vi "PH_Beamline.i attribute.vi"(0 "VI Refnum":refnum<vi>, 2 "CLASS.i attribute":T1={"GUI Refs"={"PA ok"=refnum, "MA ok"=refnum, "fs FE ok"=refnum, "ns FE ok"=refnum, "PA ED ok"=refnum, "MAS ok"=refnum, "Booster ok"=refnum, "Mirrortower ok"=refnum, "In.-Box ok"=refnum, "Compressor ok"=refnum, "Experiment LB ok"=refnum, "Experiment LL ok"=refnum, "PHELIX_Beckhoff_Watchdog"=refnum, "Shutters closed"=refnum, "uOPA ok"=refnum, "Vacuum no shotcond Comp LB"=refnum}, "Refs BL MA"=[], "Refs BL MA-IB"=[], "Refs BL fs"=[], "Refs BL PA ED"=[], "Refs BL MAS"=[], "Refs BL Boo"=[], "Refs BL ns"=[], "Refs BL Mirrortower"=[], "Refs BL Compressor"=[], "Refs BL Exp LB"=[], "Radiation Safety"={"Exp Laserbay"={"Ref Op Mode"=refnum, "Ref Laserbay evacuated"=refnum, "Tagname LB evacuated"="N/A", "Shot Mode"=0, "Laserbay evacuated?"=0, "Tagname HV room locked"="N/A", "HV room locked?"=0, "Ref HV room locked"=refnum, "Tagname bridged?"="N/A", "Ref Bridge"=refnum, "I<1E18W/cm²"=FALSE}, "Exp Laserlab"={"Ref Op Mode"=refnum, "Ref Laserlab evacuated"=refnum, "Tagname LL evacuated"="N/A", "Shot Mode"=0, "Laserlab evacuated?"=0, "Tagname bridged?"="N/A", "Ref Bridge"=refnum, "I<1E18W/cm²"=FALSE}}, "Refs BL LL"=[], "PP Igni Heating GUI Refs"=[], "PP Igni Heating Tagnames "=[], "Refs BL PA"={"undelayed Line before Shutter"=[], "undelayed Line after Shutter"=[], "before Bypass"=[], "delayed Line before Shutter"=[], "delayed Line after Shutter"=[], "before Shutter Input"=[], "after Shutter Input"=[], "Bypass"=[], "before Shutter Exit"=[], "after Shutter Exit"=[], "to MA"=[], "to Lab"=[]}, "BL"={"YLF_BL_Status"=-1, "fs_BL_Status"=-1, "fs_YLF_BL_Status"=-1, "ns_BL_Status"=-1, "PA_Input_BL_Status"=-1, "PA_UnDelay_BL_Status"=-1, "PA_Delay_BL_Status"=-1, "PA_BL_Status"=-1, "PA_Bypass_BL_Status"=-1, "PA_Exit_BL_Status"=-1, "PA_LL_BL_Status"=-1, "LL_BL_Status"=-1, "PA_MA_BL_Status"=-1, "MA_Exit_BL_Status"=-1, "MA_Z6_BL_Status"=-1, "Z6_BL_Status"=-1, "MA_LB_BL_Status"=-1, "LB_TB2_BL_Status"=-1, "PA_before_Bypass_BL_Status"=-1, "LB_TB3_BL_Status"=-1}, "State Subsystems"={"PA"=FALSE, "MA"=FALSE, "ns FE"=FALSE, "fs FE"=FALSE, "PA ED"=FALSE, "In.-Box"=FALSE, "MAS"=FALSE, "Booster"=FALSE, "Mirrortower"=FALSE, "Compressor"=FALSE, "Experiment LB"=FALSE, "Experiment LL"=FALSE, "uOPA"=FALSE}, "Status Subscriber Information"={"fs Swich YLF"={"Index of element"=-1, "Attributeset"=enum."Boolean Status Service Subscriber"}, "fs Exit Shutter"={"Index of element"=-1, "Attributeset"=enum."Boolean Status Service Subscriber"}, "ns Exit Shutter"={"Index of element"=-1, "Attributeset"=enum."Boolean Status Service Subscriber"}, "PA Input Shutter"={"Index of element"=-1, "Attributeset"=enum."Boolean Status Service Subscriber"}, "PA PC WP"={"Index of element"=-1, "Attributeset"=enum."Boolean Status Service Subscriber"}, "PA PC WP 2"={"Index of element"=-1, "Attributeset"=enum."Boolean Status Service Subscriber"}, "PA Bypass In"={"Index of element"=-1, "Attributeset"=enum."Boolean Status Service Subscriber"}, "PA Bypass Out"={"Index of element"=-1, "Attributeset"=enum."Boolean Status Service Subscriber"}, "PA CH 1"={"Index of element"=-1, "Attributeset"=enum."Boolean Status Service Subscriber"}, "PA delayed"={"Index of element"=-1, "Attributeset"=enum."Boolean Status Service Subscriber"}, "PA non delayed"={"Index of element"=-1, "Attributeset"=enum."Boolean Status Service Subscriber"}, "PA Exit Shutter"={"Index of element"=-1, "Attributeset"=enum."Boolean Status Service Subscriber"}, "PA Switch Lab"={"Index of element"=-1, "Attributeset"=enum."Boolean Status Service Subscriber"}, "PA Bridge CH Input MA"={"Index of element"=-1, "Attributeset"=enum."Boolean Status Service Subscriber"}, "MA Diffusor IB"={"Index of element"=-1, "Attributeset"=enum."Boolean Status Service Subscriber"}, "MA IB Ready"={"Index of element"=-1, "Attributeset"=enum."Boolean Status Service Subscriber"}, "MA CH 1"={"Index of element"=-1, "Attributeset"=enum."Boolean Status Service Subscriber"}, "MA CH 2"={"Index of element"=-1, "Attributeset"=enum."Boolean Status Service Subscriber"}, "MA CH 3"={"Index of element"=-1, "Attributeset"=enum."Boolean Status Service Subscriber"}, "MA CH 4"={"Index of element"=-1, "Attributeset"=enum."Boolean Status Service Subscriber"}, "MA Shutter Align Cam"={"Index of element"=-1, "Attributeset"=enum."Boolean Status Service Subscriber"}, "MA Position MM5"={"Index of element"=-1, "Attributeset"=enum."Boolean Status Service Subscriber"}, "Calorimeter Switch"={"Index of element"=-1, "Attributeset"=enum."Boolean Status Service Subscriber"}, "BL Z6 CH 9"={"Index of element"=-1, "Attributeset"=enum."Boolean Status Service Subscriber"}, "BL Z6 Beamdump"={"Index of element"=-1, "Attributeset"=enum."Boolean Status Service Subscriber"}, "BL Z6 Shutter"={"Index of element"=-1, "Attributeset"=enum."Boolean Status Service Subscriber"}, "COS Sensitivity Switch"={"Index of element"=-1, "Attributeset"=enum."Boolean Status Service Subscriber"}, "Exp LB Shutter"={"Index of element"=-1, "Attributeset"=enum."Boolean Status Service Subscriber"}, "Exp LB TB 2"={"Index of element"=-1, "Attributeset"=enum."Boolean Status Service Subscriber"}, "Exp LB TB 3"={"Index of element"=-1, "Attributeset"=enum."Boolean Status Service Subscriber"}, "PA LL Input CH"={"Index of element"=-1, "Attributeset"=enum."Boolean Status Service Subscriber"}, "PA LL Output CH"={"Index of element"=-1, "Attributeset"=enum."Boolean Status Service Subscriber"}, "LL Comp Input Shutter"={"Index of element"=-1, "Attributeset"=enum."Boolean Status Service Subscriber"}, "LL Comp Output Shutter"={"Index of element"=-1, "Attributeset"=enum."Boolean Status Service Subscriber"}, "LL Comp FF Shutter"={"Index of element"=-1, "Attributeset"=enum."Boolean Status Service Subscriber"}, "Exp LL Shutter"={"Index of element"=0, "Attributeset"=enum."Boolean Status Service Subscriber"}, "MA IM In IB"={"Index of element"=0, "Attributeset"=enum."Boolean Status Service Subscriber"}, "MA IM Out IB"={"Index of element"=0, "Attributeset"=enum."Boolean Status Service Subscriber"}, "MA DB In IB"={"Index of element"=0, "Attributeset"=enum."Boolean Status Service Subscriber"}, "MA DB Out IB"={"Index of element"=0, "Attributeset"=enum."Boolean Status Service Subscriber"}, "Exp LB Shutter Interlock"={"Index of element"=0, "Attributeset"=enum."Boolean Status Service Subscriber"}, "Exp LL Shutter Interlock"={"Index of element"=0, "Attributeset"=enum."Boolean Status Service Subscriber"}, "MM1 Force Sensor"={"Index of element"=0, "Attributeset"=enum."Boolean Status Service Subscriber"}}, "Refs BL uOPA"=[], "PA_Input_2_Beam_6PWpGUI not linked?"=FALSE, "PA_Input_Delay_6PGUI not linked?"=FALSE, "Settings"={"PA Doublepass Mode"=FALSE, "Compressor Vaccuum LB not relevant"=FALSE, "Windowshutter TB2 not relevant"=FALSE, "Windowshutter TB3 not relevant"=FALSE}} {"Radiation Safety"."Exp Laserlab"."Laserlab evacuated?" items=["no info", "LL not evacuated", "LL evacuated"]; "Radiation Safety"."Exp Laserlab"."Shot Mode" items=["no info", "no Shotmode", "Shotmode"]; "Radiation Safety"."Exp Laserbay"."HV room locked?" items=["no info", "HV room open", "HV room locked"]; "Radiation Safety"."Exp Laserbay"."Laserbay evacuated?" items=["no info", "LB not evacuated", "LB evacuated"]; "Radiation Safety"."Exp Laserbay"."Shot Mode" items=["no info", "no Shotmode", "Shotmode"]}, 3 "Action":T7(ring), 5 "error in (no error)":errorcluster) -> (14 "VI Refnum out":refnum<vi>, 16 "CLASS.i attribute out":T1={"GUI Refs"={"PA ok"=refnum, "MA ok"=refnum, "fs FE ok"=refnum, "ns FE ok"=refnum, "PA ED ok"=refnum, "MAS ok"=refnum, "Booster ok"=refnum, "Mirrortower ok"=refnum, "In.-Box ok"=refnum, "Compressor ok"=refnum, "Experiment LB ok"=refnum, "Experiment LL ok"=refnum, "PHELIX_Beckhoff_Watchdog"=refnum, "Shutters closed"=refnum, "uOPA ok"=refnum, "Vacuum no shotcond Comp LB"=refnum}, "Refs BL MA"=[], "Refs BL MA-IB"=[], "Refs BL fs"=[], "Refs BL PA ED"=[], "Refs BL MAS"=[], "Refs BL Boo"=[], "Refs BL ns"=[], "Refs BL Mirrortower"=[], "Refs BL Compressor"=[], "Refs BL Exp LB"=[], "Radiation Safety"={"Exp Laserbay"={"Ref Op Mode"=refnum, "Ref Laserbay evacuated"=refnum, "Tagname LB evacuated"="N/A", "Shot Mode"=0, "Laserbay evacuated?"=0, "Tagname HV room locked"="N/A", "HV room locked?"=0, "Ref HV room locked"=refnum, "Tagname bridged?"="N/A", "Ref Bridge"=refnum, "I<1E18W/cm²"=FALSE}, "Exp Laserlab"={"Ref Op Mode"=refnum, "Ref Laserlab evacuated"=refnum, "Tagname LL evacuated"="N/A", "Shot Mode"=0, "Laserlab evacuated?"=0, "Tagname bridged?"="N/A", "Ref Bridge"=refnum, "I<1E18W/cm²"=FALSE}}, "Refs BL LL"=[], "PP Igni Heating GUI Refs"=[], "PP Igni Heating Tagnames "=[], "Refs BL PA"={"undelayed Line before Shutter"=[], "undelayed Line after Shutter"=[], "before Bypass"=[], "delayed Line before Shutter"=[], "delayed Line after Shutter"=[], "before Shutter Input"=[], "after Shutter Input"=[], "Bypass"=[], "before Shutter Exit"=[], "after Shutter Exit"=[], "to MA"=[], "to Lab"=[]}, "BL"={"YLF_BL_Status"=-1, "fs_BL_Status"=-1, "fs_YLF_BL_Status"=-1, "ns_BL_Status"=-1, "PA_Input_BL_Status"=-1, "PA_UnDelay_BL_Status"=-1, "PA_Delay_BL_Status"=-1, "PA_BL_Status"=-1, "PA_Bypass_BL_Status"=-1, "PA_Exit_BL_Status"=-1, "PA_LL_BL_Status"=-1, "LL_BL_Status"=-1, "PA_MA_BL_Status"=-1, "MA_Exit_BL_Status"=-1, "MA_Z6_BL_Status"=-1, "Z6_BL_Status"=-1, "MA_LB_BL_Status"=-1, "LB_TB2_BL_Status"=-1, "PA_before_Bypass_BL_Status"=-1, "LB_TB3_BL_Status"=-1}, "State Subsystems"={"PA"=FALSE, "MA"=FALSE, "ns FE"=FALSE, "fs FE"=FALSE, "PA ED"=FALSE, "In.-Box"=FALSE, "MAS"=FALSE, "Booster"=FALSE, "Mirrortower"=FALSE, "Compressor"=FALSE, "Experiment LB"=FALSE, "Experiment LL"=FALSE, "uOPA"=FALSE}, "Status Subscriber Information"={"fs Swich YLF"={"Index of element"=-1, "Attributeset"=enum."Boolean Status Service Subscriber"}, "fs Exit Shutter"={"Index of element"=-1, "Attributeset"=enum."Boolean Status Service Subscriber"}, "ns Exit Shutter"={"Index of element"=-1, "Attributeset"=enum."Boolean Status Service Subscriber"}, "PA Input Shutter"={"Index of element"=-1, "Attributeset"=enum."Boolean Status Service Subscriber"}, "PA PC WP"={"Index of element"=-1, "Attributeset"=enum."Boolean Status Service Subscriber"}, "PA PC WP 2"={"Index of element"=-1, "Attributeset"=enum."Boolean Status Service Subscriber"}, "PA Bypass In"={"Index of element"=-1, "Attributeset"=enum."Boolean Status Service Subscriber"}, "PA Bypass Out"={"Index of element"=-1, "Attributeset"=enum."Boolean Status Service Subscriber"}, "PA CH 1"={"Index of element"=-1, "Attributeset"=enum."Boolean Status Service Subscriber"}, "PA delayed"={"Index of element"=-1, "Attributeset"=enum."Boolean Status Service Subscriber"}, "PA non delayed"={"Index of element"=-1, "Attributeset"=enum."Boolean Status Service Subscriber"}, "PA Exit Shutter"={"Index of element"=-1, "Attributeset"=enum."Boolean Status Service Subscriber"}, "PA Switch Lab"={"Index of element"=-1, "Attributeset"=enum."Boolean Status Service Subscriber"}, "PA Bridge CH Input MA"={"Index of element"=-1, "Attributeset"=enum."Boolean Status Service Subscriber"}, "MA Diffusor IB"={"Index of element"=-1, "Attributeset"=enum."Boolean Status Service Subscriber"}, "MA IB Ready"={"Index of element"=-1, "Attributeset"=enum."Boolean Status Service Subscriber"}, "MA CH 1"={"Index of element"=-1, "Attributeset"=enum."Boolean Status Service Subscriber"}, "MA CH 2"={"Index of element"=-1, "Attributeset"=enum."Boolean Status Service Subscriber"}, "MA CH 3"={"Index of element"=-1, "Attributeset"=enum."Boolean Status Service Subscriber"}, "MA CH 4"={"Index of element"=-1, "Attributeset"=enum."Boolean Status Service Subscriber"}, "MA Shutter Align Cam"={"Index of element"=-1, "Attributeset"=enum."Boolean Status Service Subscriber"}, "MA Position MM5"={"Index of element"=-1, "Attributeset"=enum."Boolean Status Service Subscriber"}, "Calorimeter Switch"={"Index of element"=-1, "Attributeset"=enum."Boolean Status Service Subscriber"}, "BL Z6 CH 9"={"Index of element"=-1, "Attributeset"=enum."Boolean Status Service Subscriber"}, "BL Z6 Beamdump"={"Index of element"=-1, "Attributeset"=enum."Boolean Status Service Subscriber"}, "BL Z6 Shutter"={"Index of element"=-1, "Attributeset"=enum."Boolean Status Service Subscriber"}, "COS Sensitivity Switch"={"Index of element"=-1, "Attributeset"=enum."Boolean Status Service Subscriber"}, "Exp LB Shutter"={"Index of element"=-1, "Attributeset"=enum."Boolean Status Service Subscriber"}, "Exp LB TB 2"={"Index of element"=-1, "Attributeset"=enum."Boolean Status Service Subscriber"}, "Exp LB TB 3"={"Index of element"=-1, "Attributeset"=enum."Boolean Status Service Subscriber"}, "PA LL Input CH"={"Index of element"=-1, "Attributeset"=enum."Boolean Status Service Subscriber"}, "PA LL Output CH"={"Index of element"=-1, "Attributeset"=enum."Boolean Status Service Subscriber"}, "LL Comp Input Shutter"={"Index of element"=-1, "Attributeset"=enum."Boolean Status Service Subscriber"}, "LL Comp Output Shutter"={"Index of element"=-1, "Attributeset"=enum."Boolean Status Service Subscriber"}, "LL Comp FF Shutter"={"Index of element"=-1, "Attributeset"=enum."Boolean Status Service Subscriber"}, "Exp LL Shutter"={"Index of element"=0, "Attributeset"=enum."Boolean Status Service Subscriber"}, "MA IM In IB"={"Index of element"=0, "Attributeset"=enum."Boolean Status Service Subscriber"}, "MA IM Out IB"={"Index of element"=0, "Attributeset"=enum."Boolean Status Service Subscriber"}, "MA DB In IB"={"Index of element"=0, "Attributeset"=enum."Boolean Status Service Subscriber"}, "MA DB Out IB"={"Index of element"=0, "Attributeset"=enum."Boolean Status Service Subscriber"}, "Exp LB Shutter Interlock"={"Index of element"=0, "Attributeset"=enum."Boolean Status Service Subscriber"}, "Exp LL Shutter Interlock"={"Index of element"=0, "Attributeset"=enum."Boolean Status Service Subscriber"}, "MM1 Force Sensor"={"Index of element"=0, "Attributeset"=enum."Boolean Status Service Subscriber"}}, "Refs BL uOPA"=[], "PA_Input_2_Beam_6PWpGUI not linked?"=FALSE, "PA_Input_Delay_6PGUI not linked?"=FALSE, "Settings"={"PA Doublepass Mode"=FALSE, "Compressor Vaccuum LB not relevant"=FALSE, "Windowshutter TB2 not relevant"=FALSE, "Windowshutter TB3 not relevant"=FALSE}} {"Radiation Safety"."Exp Laserlab"."Laserlab evacuated?" items=["no info", "LL not evacuated", "LL evacuated"]; "Radiation Safety"."Exp Laserlab"."Shot Mode" items=["no info", "no Shotmode", "Shotmode"]; "Radiation Safety"."Exp Laserbay"."HV room locked?" items=["no info", "HV room open", "HV room locked"]; "Radiation Safety"."Exp Laserbay"."Laserbay evacuated?" items=["no info", "LB not evacuated", "LB evacuated"]; "Radiation Safety"."Exp Laserbay"."Shot Mode" items=["no info", "no Shotmode", "Shotmode"]}, 19 "error out":errorcluster)   [LabVIEW 2014, in "PH_Beamline.lvlib"]
doc: "This is a so-called functional global variable. It manages the access to a global variable in a thread-safe way. \n\nHere the attribute data of all instances of THIS class are stored. This is done for performance reasons.\n\nLicense Agreement for this software:\n\nCopyright (C)\nGesellschaft für Schwerionenforschung, GSI\nPlanckstr. 1\n64291 Darmstadt\nGermany\n\nContact: D.Beck@gsi.de \n\nThis program is free software; you can redistribute it and/or modify it under the terms of the GNU General Public License as published by the Free Software Foundation; either version 2 of the license, or (at your option) any later version.\n\nThis program is distributed in the hope that it will be useful, but WITHOUT ANY WARRANTY; without even the implied warranty of MERCHANTABILITY or FITNESS FOR A PARTICULAR PURPOSE. See the GNU General License for more details (http://www.gnu.org).\n\nGesellschaft für Schwerionenforschung, GSI\nPlanckstr. 1, 64291 Darmstadt, Germany\nFor all questions and ideas contact: M.Richter@gsi.de, H.Brand@gsi.de or D.Beck@gsi.de.\nLast update: 17-JUN-2004"
uses:
  PH_Beamline.lvlib
  PH_Beamline.i attribute.ctl
  PH_Beamline.Operation Mode.ctl
  PH_Beamline.Status Subscriber Information.ctl
  PH_BL-Master/PH_BL-Master.Status Subscriber Information.ctl
  PH_BL-Master/PH_BL-Master.Attribute Set.ctl
  PH_Beamline_Chief/PH_Beamline_Chief.Settings.ctl
  CS_Core/CSSystem/CoreDefs/CoreDefs.error_type.ctl
  CS_Core/CSSystem/CoreLib/CoreLib.lvlib
  PH_BL-Master/PH_BL-Master.lvlib
  PH_Beamline_Chief/PH_Beamline_Chief.lvlib
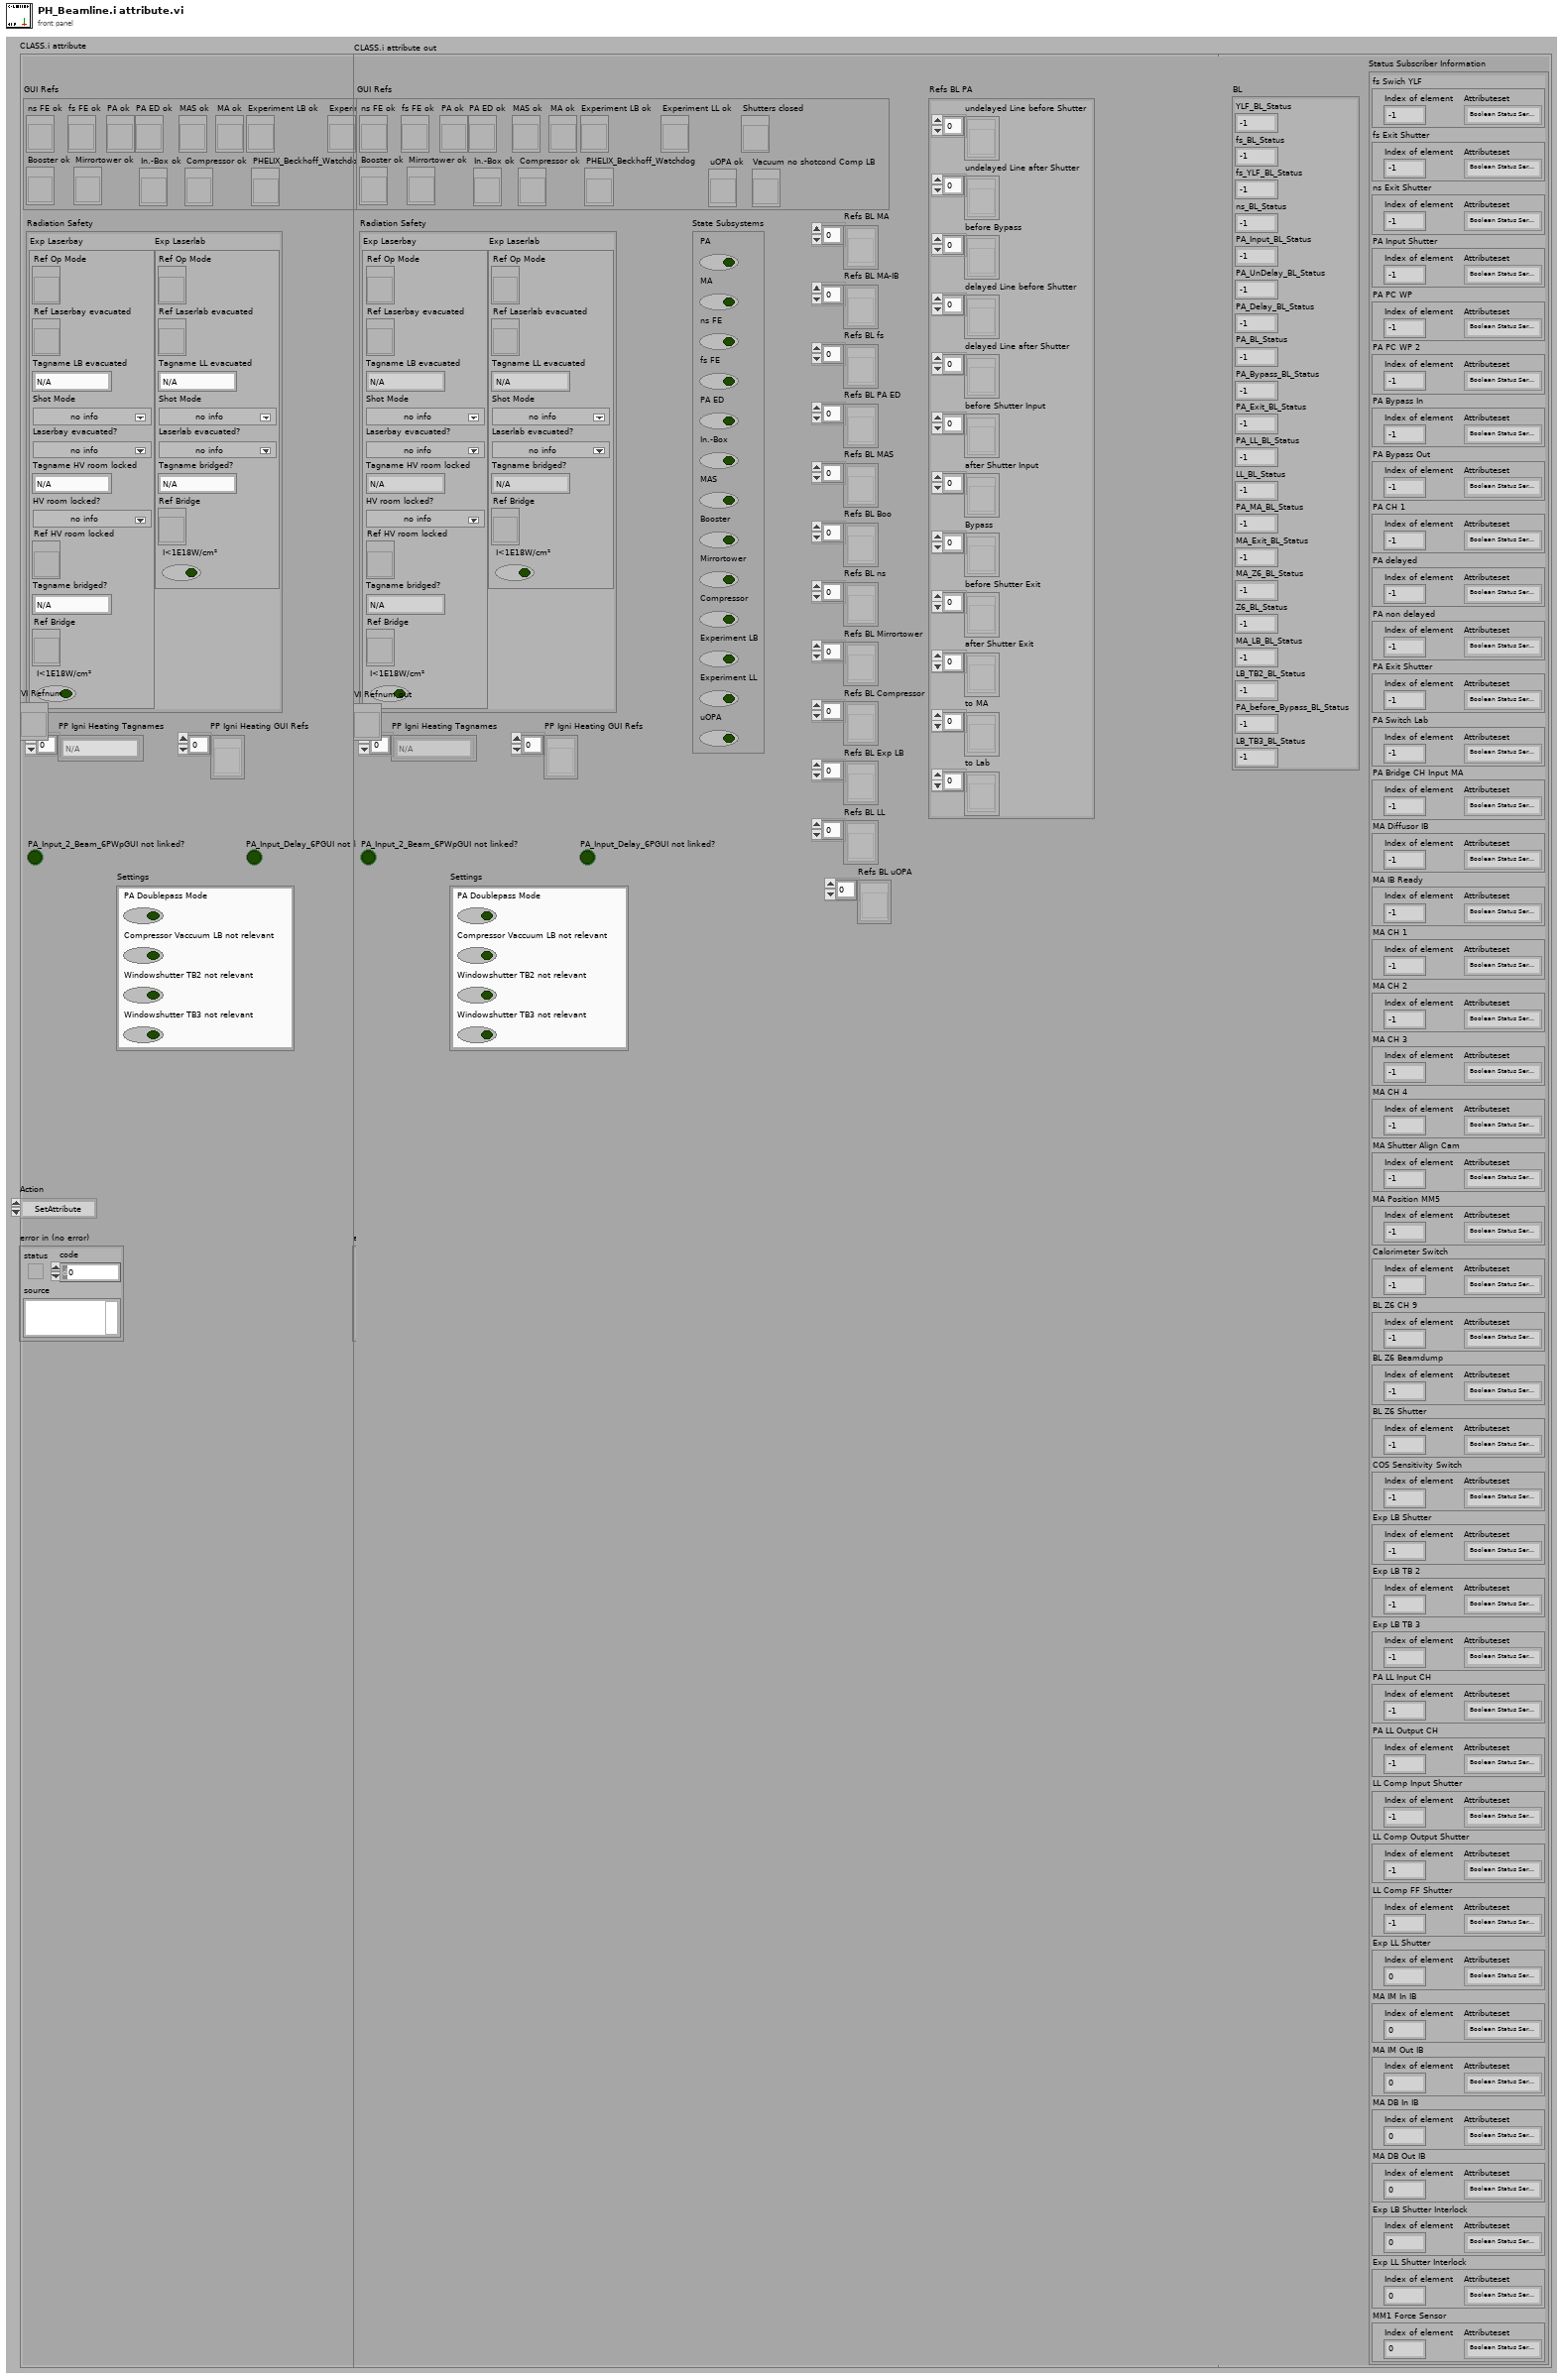
[diagram p1: front panel]
types:
  T1 = typedef "PH_Beamline.lvlib/PH_Beamline.i attribute.ctl" = cluster{"GUI Refs":cluster{"PA ok":refnum<vi>, "MA ok":refnum<vi>, "fs FE ok":refnum<vi>, "ns FE ok":refnum<vi>, "PA ED ok":refnum<vi>, "MAS ok":refnum<vi>, "Booster ok":refnum<vi>, "Mirrortower ok":refnum<vi>, "In.-Box ok":refnum<vi>, "Compressor ok":refnum<vi>, "Experiment LB ok":refnum<vi>, "Experiment LL ok":refnum<vi>, "PHELIX_Beckhoff_Watchdog":refnum<vi>, "Shutters closed":refnum<vi>, "uOPA ok":refnum<vi>, "Vacuum no shotcond Comp LB":refnum<vi>}, "Refs BL MA":refnum<vi>[], "Refs BL MA-IB":refnum<vi>[], "Refs BL fs":refnum<vi>[], "Refs BL PA ED":refnum<vi>[], "Refs BL MAS":refnum<vi>[], "Refs BL Boo":refnum<vi>[], "Refs BL ns":refnum<vi>[], "Refs BL Mirrortower":refnum<vi>[], "Refs BL Compressor":refnum<vi>[], "Refs BL Exp LB":refnum<vi>[], "Radiation Safety":cluster{"Exp Laserbay":cluster{"Ref Op Mode":refnum<vi>, "Ref Laserbay evacuated":refnum<vi>, "Tagname LB evacuated":string, "Shot Mode":T2, "Laserbay evacuated?":i32, "Tagname HV room locked":string, "HV room locked?":i32, "Ref HV room locked":refnum<vi>, "Tagname bridged?":string, "Ref Bridge":refnum<vi>, "I<1E18W/cm²":bool}, "Exp Laserlab":cluster{"Ref Op Mode":refnum<vi>, "Ref Laserlab evacuated":refnum<vi>, "Tagname LL evacuated":string, "Shot Mode":T2, "Laserlab evacuated?":i32, "Tagname bridged?":string, "Ref Bridge":refnum<vi>, "I<1E18W/cm²":bool}}, "Refs BL LL":refnum<vi>[], "PP Igni Heating GUI Refs":refnum<vi>[], "PP Igni Heating Tagnames ":string[], "Refs BL PA":cluster{"undelayed Line before Shutter":refnum<vi>[], "undelayed Line after Shutter":refnum<vi>[], "before Bypass":refnum<vi>[], "delayed Line before Shutter":refnum<vi>[], "delayed Line after Shutter":refnum<vi>[], "before Shutter Input":refnum<vi>[], "after Shutter Input":refnum<vi>[], "Bypass":refnum<vi>[], "before Shutter Exit":refnum<vi>[], "after Shutter Exit":refnum<vi>[], "to MA":refnum<vi>[], "to Lab":refnum<vi>[]}, "BL":cluster{"YLF_BL_Status":i32, "fs_BL_Status":i32, "fs_YLF_BL_Status":i32, "ns_BL_Status":i32, "PA_Input_BL_Status":i32, "PA_UnDelay_BL_Status":i32, "PA_Delay_BL_Status":i32, "PA_BL_Status":i32, "PA_Bypass_BL_Status":i32, "PA_Exit_BL_Status":i32, "PA_LL_BL_Status":i32, "LL_BL_Status":i32, "PA_MA_BL_Status":i32, "MA_Exit_BL_Status":i32, "MA_Z6_BL_Status":i32, "Z6_BL_Status":i32, "MA_LB_BL_Status":i32, "LB_TB2_BL_Status":i32, "PA_before_Bypass_BL_Status":i32, "LB_TB3_BL_Status":i32}, "State Subsystems":cluster{"PA":bool, "MA":bool, "ns FE":bool, "fs FE":bool, "PA ED":bool, "In.-Box":bool, "MAS":bool, "Booster":bool, "Mirrortower":bool, "Compressor":bool, "Experiment LB":bool, "Experiment LL":bool, "uOPA":bool}, "Status Subscriber Information":T3, "Refs BL uOPA":refnum<vi>[], "PA_Input_2_Beam_6PWpGUI not linked?":bool, "PA_Input_Delay_6PGUI not linked?":bool, "Settings":T6}
  T2 = typedef "PH_Beamline.lvlib/PH_Beamline.Operation Mode.ctl" = i32
  T3 = typedef "PH_Beamline.lvlib/PH_Beamline.Status Subscriber Information.ctl" = cluster{"fs Swich YLF":T4, "fs Exit Shutter":T4, "ns Exit Shutter":T4, "PA Input Shutter":T4, "PA PC WP":T4, "PA PC WP 2":T4, "PA Bypass In":T4, "PA Bypass Out":T4, "PA CH 1":T4, "PA delayed":T4, "PA non delayed":T4, "PA Exit Shutter":T4, "PA Switch Lab":T4, "PA Bridge CH Input MA":T4, "MA Diffusor IB":T4, "MA IB Ready":T4, "MA CH 1":T4, "MA CH 2":T4, "MA CH 3":T4, "MA CH 4":T4, "MA Shutter Align Cam":T4, "MA Position MM5":T4, "Calorimeter Switch":T4, "BL Z6 CH 9":T4, "BL Z6 Beamdump":T4, "BL Z6 Shutter":T4, "COS Sensitivity Switch":T4, "Exp LB Shutter":T4, "Exp LB TB 2":T4, "Exp LB TB 3":T4, "PA LL Input CH":T4, "PA LL Output CH":T4, "LL Comp Input Shutter":T4, "LL Comp Output Shutter":T4, "LL Comp FF Shutter":T4, "Exp LL Shutter":T4, "MA IM In IB":T4, "MA IM Out IB":T4, "MA DB In IB":T4, "MA DB Out IB":T4, "Exp LB Shutter Interlock":T4, "Exp LL Shutter Interlock":T4, "MM1 Force Sensor":T4}
  T4 = typedef "PH_BL-Master.lvlib/PH_BL-Master.Status Subscriber Information.ctl" = cluster{"Index of element":i32, "Attributeset":T5}
  T5 = typedef "PH_BL-Master.lvlib/PH_BL-Master.Attribute Set.ctl" = enum16{"Boolean Status Service Subscriber", "Picture Status Service Subscriber"}
  T6 = typedef "PH_Beamline_Chief.lvlib/PH_Beamline_Chief.Settings.ctl" = cluster{"PA Doublepass Mode":bool, "Compressor Vaccuum LB not relevant":bool, "Windowshutter TB2 not relevant":bool, "Windowshutter TB3 not relevant":bool}
  T7 = enum16{"SetAttribute", "GetAttribute", "CreateAttribute", "DestroyAttribute", "DestroyAllAtributes"}
  T8 = typedef "CoreDefs.error_type.ctl" = enum16{"no error", "can't load process", "can't unload process", "process does not exist", "can't install process", "can't remove process", "unknown function", "time out", "can't execute function", "duplicate queue name", "super not found", "caller queue invalid", "can't ping process", "unknown error", "VISA Error", "VISA timeout", "GPIB timeout", "GPIB error", "communication error", "data type mismatch", "can't read data from OPC server", "can't write data to OPC server", "OET error", "function not implemented", "process already exists", "invalid Shared Variable name", "error writing Shared Variable", "error reading Shared Variable", "invalid client name", "corrupt database", "unknown class", "call not authorized", "parameter out of range", "OET timeout: can't get data to modify", "invalid queue name", "requested operation incompatible with current state", "event undefined", "event disabled", "state undefined", "caller is not a friend", "EventBuilder: bad eventID", "EventBuilder: no DAQ devices", "a thread must not stop itself", "UNUSED ELEMENT4", "DiscArchiver: eventData incomplete", "DiscArchiver: eventData does not belong to run", "DiscArchiver: can't open file", "DiscArchiver: can't write to file", "DiscArchiver: available disc space low", "can't acquire semaphore", "error reading data from database", "notifier object is not existing", "can't register process", "can't unregister process", "illegal event type", "object disabled", "object already exists", "can't change state", "Instrument not found", "no connection to remote node", "invalid reference", "N/A", "UNUSED ELEMENT 1", "element not found", "illegal TCP/IP connection detected", "object does not exist", "invalid access ID", "unknown CS system", "invalid privilige", "unsupported data type", "unsupported server type", "IO server already exists", "Shared Variable already exists"}
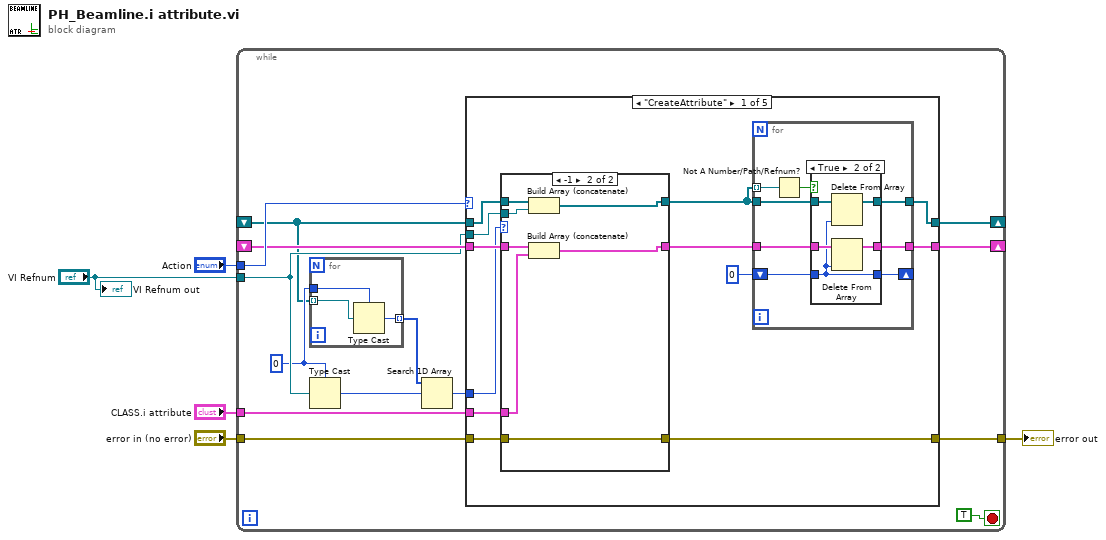
[diagram p0: block diagram]
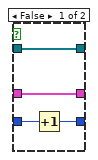
[diagram p2: hidden frame]
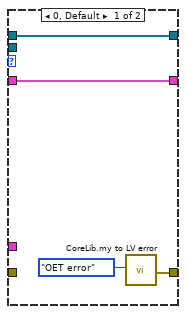
[diagram p3: hidden frame]
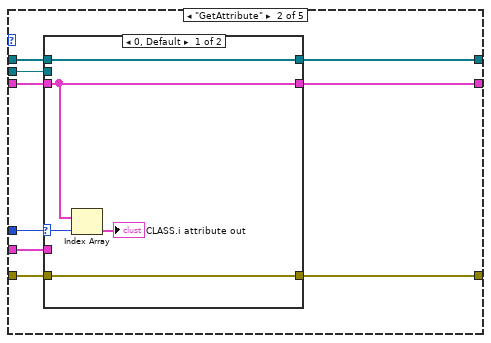
[diagram p4: hidden frame]
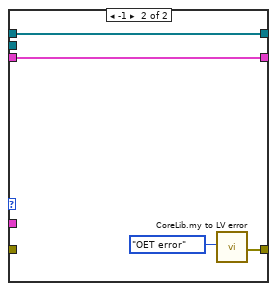
[diagram p5: hidden frame]
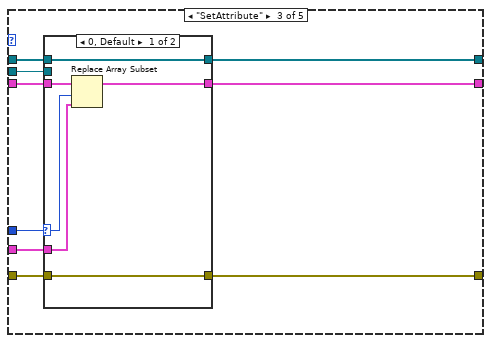
[diagram p6: hidden frame]
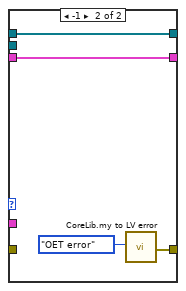
[diagram p7: hidden frame]
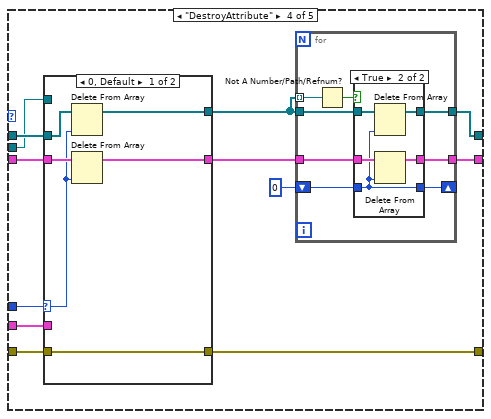
[diagram p8: hidden frame]
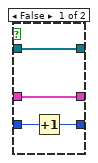
[diagram p9: hidden frame]
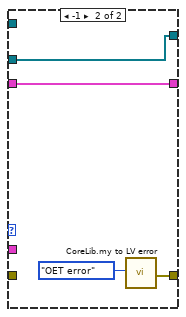
[diagram p10: hidden frame]
diagram:
  n1 = while {
    shift-right: [w13] -> _
    shift-left: _ -> [w14]
    tunnel: "Action" -> [w18]
    shift-right: [w15] -> _
    shift-left: _ -> [w6]
    tunnel: "error in (no error)" -> [w17]
    tunnel: [w16] -> w3
    tunnel: "CLASS.i attribute" -> [w12]
    tunnel: "VI Refnum" -> [w9]
    stop <- TRUE stop-if-true
    w8 = 0
    n2 = for {
      tunnel: w8 -> [w22]
      tunnel: [w21] -> w7 mode=indexing
      tunnel: w6 -> [w20] mode=indexing
      n3 = Type Cast(type=w22, x=w20) -> (*(type *) &x=w21:i32)
    }
    n4 = Type Cast(type=w8, x=w9) -> (*(type *) &x=w10:i32)
    n5 = Search 1D Array(1D array=w7, element=w10) -> (index of element=w11:i32)  [unwired: 1 in]
    n6 = case shown="\"CreateAttribute\"" w18 {
      tunnel: w6 -> [w32 w69 w87 w109 _]
      tunnel: w9 -> [w31 w67 w85 w108 _]
      tunnel: w17 -> [w34 w71 w89 w111 w139]
      tunnel: [w33 w70 w88 w110 w139] -> w16
      tunnel: [w26 w68 w86 w103 _] -> w15
      tunnel: w14 -> [w30 w66 w84 w107 _]
      tunnel: [w25 w65 w83 w101 _] -> w13
      tunnel: w12 -> [w29 w64 w82 w106 _]
      tunnel: w11 -> [w28 w63 w81 w105 _]
      frame "CreateAttribute" {
        n7 = case shown="-1" w28 {
          tunnel: w34 -> [_ w62]
          tunnel: [w54 w62] -> w33
          tunnel: w32 -> [w53 w61]
          tunnel: [w53 w60] -> w24
          tunnel: w31 -> [_ w59]
          tunnel: w30 -> [w52 w58]
          tunnel: [w52 w57] -> w23
          tunnel: w29 -> [_ w56]
          frame 0, Default {
            n8 = call "CoreLib.my to LV error.vi"("ErrorTypes"=CoreDefs.error_type."OET error") -> ("myErrorCluster"=w54:errorcluster)  [unwired: 17 in, 1 out]
          }
          frame -1 {
            n9 = Build Array (concatenate)(w61, w59) -> (w60:refnum<vi>[])
            n10 = Build Array (concatenate)(w58, w56) -> (w57:T1[])
          }
        }
        n11 = for {
          tunnel: w24 -> [w39]
          tunnel: [w38] -> w26
          tunnel: [w42] -> w25
          tunnel: w23 -> [w41]
          tunnel: w24 -> [w37] mode=indexing
          shift-right: [w36] -> _
          shift-left: 0 -> [w35]
          n12 = Not A Number/Path/Refnum?(number/path/refnum=w37) -> (NaN/Path/Refnum?=w40:bool)
          n13 = case shown="True" w40 {
            tunnel: [w46 w51] -> w42
            tunnel: w41 -> [w46 w50]
            tunnel: [w45 w48] -> w38
            tunnel: w39 -> [w45 w49]
            tunnel: w35 -> [w44 w47]
            tunnel: [w43 w47] -> w36
            frame False {
              n14 = Increment(x=w44) -> (x+1=w43:i32)
            }
            frame True {
              n15 = Delete From Array(array=w49, index=w47) -> (array with subset deleted=w48:refnum<vi>[])  [unwired: 1 in, 1 out]
              n16 = Delete From Array(array=w50, index=w47) -> (array with subset deleted=w51:T1[])  [unwired: 1 in, 1 out]
            }
          }
        }
      }
      frame "GetAttribute" {
        n17 = case shown="0, Default" w63 {
          selector: w63 -> [w74 _]
          tunnel: w71 -> [w76 _]
          tunnel: [w76 w79] -> w70
          tunnel: w69 -> [w75 w78]
          tunnel: [w75 w78] -> w68
          tunnel: w67 -> [_ _]
          tunnel: w66 -> [w73 w77]
          tunnel: [w73 w77] -> w65
          tunnel: w64 -> [_ _]
          frame 0, Default {
            n18 = Index Array(array=w73, index=w74) -> (element=→"CLASS.i attribute out":T1)
          }
          frame -1 {
            n19 = call "CoreLib.my to LV error.vi"("ErrorTypes"=CoreDefs.error_type."OET error") -> ("myErrorCluster"=w79:errorcluster)  [unwired: 17 in, 1 out]
          }
        }
      }
      frame "SetAttribute" {
        n20 = case shown="0, Default" w81 {
          selector: w81 -> [w91 _]
          tunnel: w89 -> [w95 _]
          tunnel: [w95 w98] -> w88
          tunnel: w87 -> [w94 w97]
          tunnel: [w94 w97] -> w86
          tunnel: w85 -> [_ _]
          tunnel: w84 -> [w93 w96]
          tunnel: [w92 w96] -> w83
          tunnel: w82 -> [w90 _]
          frame 0, Default {
            n21 = Replace Array Subset(array=w93, new element=w90, index=w91) -> (w92:T1[])
          }
          frame -1 {
            n22 = call "CoreLib.my to LV error.vi"("ErrorTypes"=CoreDefs.error_type."OET error") -> ("myErrorCluster"=w98:errorcluster)  [unwired: 17 in, 1 out]
          }
        }
      }
      frame "DestroyAttribute" {
        n23 = case shown="0, Default" w105 {
          selector: w105 -> [w130 _]
          tunnel: w111 -> [w134 _]
          tunnel: [w134 w137] -> w110
          tunnel: w109 -> [w133 w136]
          tunnel: [w132 w136] -> w102
          tunnel: w108 -> [_ _]
          tunnel: w107 -> [w131 w135]
          tunnel: [w129 w135] -> w100
          tunnel: w106 -> [_ _]
          frame 0, Default {
            n24 = Delete From Array(array=w133, index=w130) -> (array with subset deleted=w132:refnum<vi>[])  [unwired: 1 in, 1 out]
            n25 = Delete From Array(array=w131, index=w130) -> (array with subset deleted=w129:T1[])  [unwired: 1 in, 1 out]
          }
          frame -1 {
            n26 = call "CoreLib.my to LV error.vi"("ErrorTypes"=CoreDefs.error_type."OET error") -> ("myErrorCluster"=w137:errorcluster)  [unwired: 17 in, 1 out]
          }
        }
        n27 = for {
          tunnel: w102 -> [w116]
          tunnel: [w115] -> w103
          tunnel: [w119] -> w101
          tunnel: w100 -> [w118]
          tunnel: w102 -> [w114] mode=indexing
          shift-right: [w113] -> _
          shift-left: 0 -> [w112]
          n28 = Not A Number/Path/Refnum?(number/path/refnum=w114) -> (NaN/Path/Refnum?=w117:bool)
          n29 = case shown="True" w117 {
            tunnel: [w123 w128] -> w119
            tunnel: w118 -> [w123 w127]
            tunnel: [w122 w125] -> w115
            tunnel: w116 -> [w122 w126]
            tunnel: w112 -> [w121 w124]
            tunnel: [w120 w124] -> w113
            frame False {
              n30 = Increment(x=w121) -> (x+1=w120:i32)
            }
            frame True {
              n31 = Delete From Array(array=w126, index=w124) -> (array with subset deleted=w125:refnum<vi>[])  [unwired: 1 in, 1 out]
              n32 = Delete From Array(array=w127, index=w124) -> (array with subset deleted=w128:T1[])  [unwired: 1 in, 1 out]
            }
          }
        }
      }
      frame "DestroyAllAtributes" {
      }
    }
  }
  "error out" <- w3
  "VI Refnum out" <- "VI Refnum"
